vi "Labview_Voltage_Logger_All_Sensors.vi"() -> ()   [LabVIEW 2018]
doc: "I. Description:\nThis example demonstrates how to input a single Current reading on an Analog Input Channel.\n\nII. Instructions for Running:\n1. Select the Physical Channel to correspond to where your signal is input on the DAQ Device.\n2. Enter the Minimum and Maximum Current Range.\nNote: For better accuracy try to match the Input Range to the expected current level of the measured signal.\n3. Enter in the parameters of your current shunt resistor. The shunt resistor location will usually be \"External\" unless you are using an SCXI current input terminal block or SCC current input module. The shunt resistor value must correspond to the shunt resistor that you are using, and is specified in ohms. If you are using an SCXI current input terminal block or SCC current input module, you must select \"Internal\" for the shunt resistor location. \n \nIII. Block Diagram Steps:\n1. Create an Analog Input Current Channel.\n2. Use the Read VI to Acquire 1 Sample on 1 Channel on the Data Acquisition Card. \n3. Call the Clear Task VI to clear the Task. \n4. Use the popup dialog box to display an error if any. \n\nIV. I/O Connections Overview:\nMake sure your signal input terminal matches the physical channel I/O control. If you are using an external shunt resistor, make sure to hook it up in parallel with the current signal you are trying to measure."
uses:
  <vilib>/Utility/error.llb/DialogType.ctl
  <vilib>/DAQmx/read.llb/DAQmx Read (Analog DBL 1Chan 1Samp).vi
  <vilib>/DAQmx/create/channels.llb/DAQmx Create Channel (AI-Voltage-Basic).vi
  <vilib>/DAQmx/miscellaneous.llb/DAQmx Fill In Error Info.vi
panel:
  out "date/time string":string
  in  "input terminal config":i32(ring)=10106 items=["Default"=-1, "RSE"=10083, "NRSE"=10078, "Differential"=10106, "Pseudodifferential"=12529]
  in  "Durafet & DirecTemp  Spreadsheet":bool
  in  "MSFET 208 Spreadsheet":bool
  in  "MSFET 202  Spreadsheet":bool
  in  "Physical Channel 6":tag="Dev1/ai2"
  out "Ch. 3":dbl(graph)=1.4978875216444314
  in  "?":bool
  out "MS 208 Temp":dbl=nan
  out "MS 202 temp":dbl=nan
  in  "?":bool
  in  "Physical Channel 11":tag="Dev1/ai7"
  out "Ch. 8":dbl(graph)=0.8511440075618667
  in  "?":bool
  in  "Physical Channel 10":tag="Dev1/ai6"
  out "Ch. 7":dbl(graph)=0.7196247243240289
  out "DF Temp":dbl=64.59754863433032 format="%.5f"
  out "pH 3":dbl=5.329485940181883 format="%.5f"
  out "pH 2":dbl=nan format="%.5f"
  out "pH":dbl=nan format="%.5f"
  in  "Sensor in":string(combo)="DuraFET"
  out "Std dev":dbl=0.023605620391285137 format="%.5f"
  out "Voltage":dbl=0.16091888454936415 format="%.5f"
  out "Std dev":dbl=0.0006550750816912838 format="%.5f"
  out "Voltage":dbl=0.12185794600876779 format="%.5f"
  in  "?":bool
  in  "Physical Channel 9":tag="Dev1/ai5"
  out "Ch. 6":dbl(graph)=0.19601783529867856
  in  "?":bool=TRUE
  in  "?":tag="Dev1/ai4"
  out "Plot":dbl(graph)=0.12072360061828691
  out "DirecTemp":string="23.310"
  out "Ch. 4":dbl(graph)=1.780653601790566
  in  "Sensor 2":string(combo)="MSFET 208"
  in  "Sensor":string(combo)="MSFET 202"
  in  "MSFET 208":path=path "C:/Users/Garrett/Google Drive/Documents/Martz Lab/Sensors/pH_Voltages208.csv"
  in  "?":bool
  out "Run Number":i32=15
  out "Ch. 2":dbl(graph)=1.7425130298801692
  out "Ch. 1":dbl(graph)=1.5015042938814973
  in  "MSFET 202":path=path "C:/Users/Garrett/Google Drive/Documents/Martz Lab/Sensors/pH_Voltages202.csv"
  in  "# for avg.":i32=10
  in  "?":bool
  in  "?":bool
  in  "?":bool
  in  "Physical Channel 7":tag="Dev1/ai3"
  out "Std dev":dbl=nan format="%.5f"
  out "Voltage":dbl=nan format="%.5f"
  out "Std dev":dbl=nan format="%.5f"
  out "Std dev":dbl=nan format="%.5f"
  out "Std dev":dbl=nan format="%.6f"
  in  "Max Voltage":dbl=1.0 format="%0.3f"
  in  "Min Voltage":dbl=-1.0 format="%0.3f"
  in  "Physical Channel 5":tag="Dev1/ai1"
  out "Voltage":dbl=nan format="%.5f"
  out "Voltage":dbl=nan format="%.5f"
  in  "Physical Channel 4":tag="Dev1/ai0"
  out "Voltage":dbl=nan format="%.6f"
  in  "For DuraFET":path=path "C:/Users/Garrett/Google Drive/Documents/Martz Lab/Sensors/pH_VoltagesDurafet.csv"
  # "OUTPUTS"
  # "INPUTS"
  # "Min Voltage"
  # "Max Voltage"
  # "Amount of meas. to avg. for data point"
  # "MSFET 202"
  # "MSFET 208"
  # "REF Voltage"
  # "pH Voltage"
  # "REF Voltage"
  # "pH Voltage"
  # "pH Voltage"
  # "Temp Voltage"
  # "Temp Voltage"
  # "Temp Voltage"
  # "+ AI0 -"
  # "+ AI1 -"
  # "+ AI2 -"
  # "+ AI3 -"
  # "+ AI4 -"
  # "+ AI5-"
  # "+ AI6-"
  # "+ AI7-"
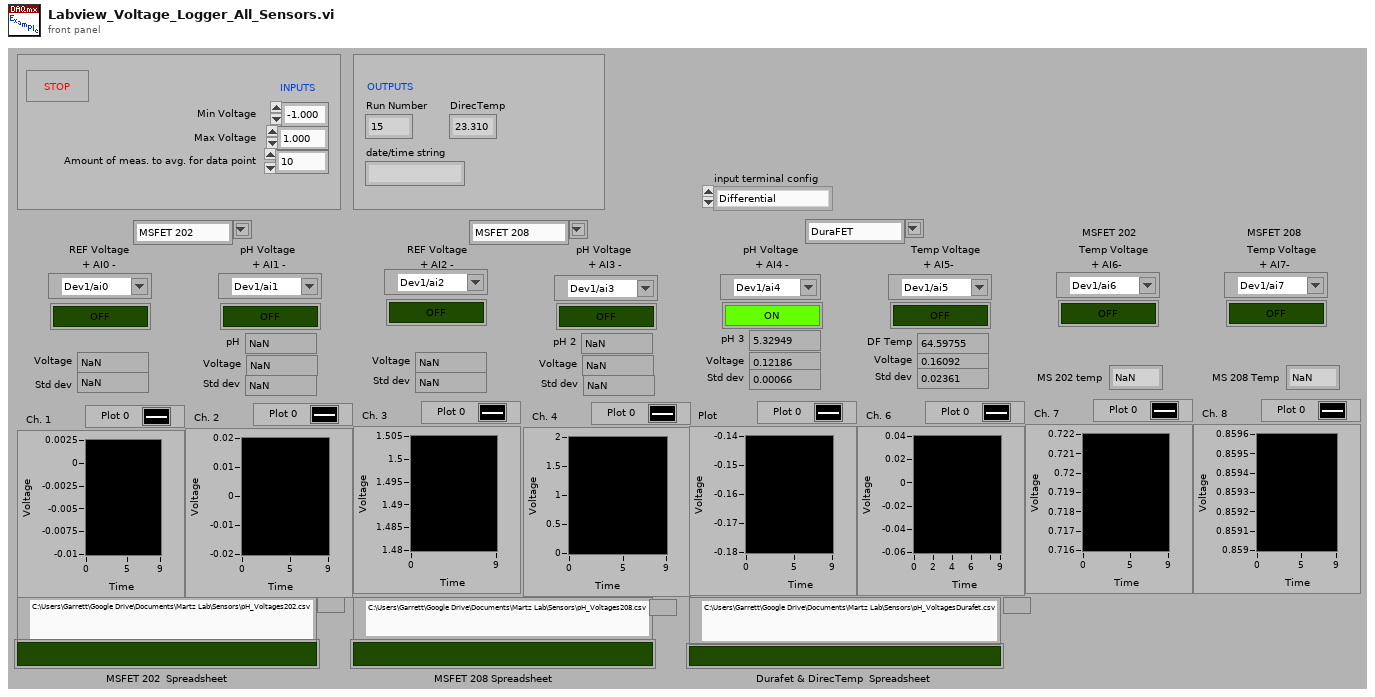
[diagram p1: front panel]
types:
  T1 = typedef "DialogType.ctl" = u16
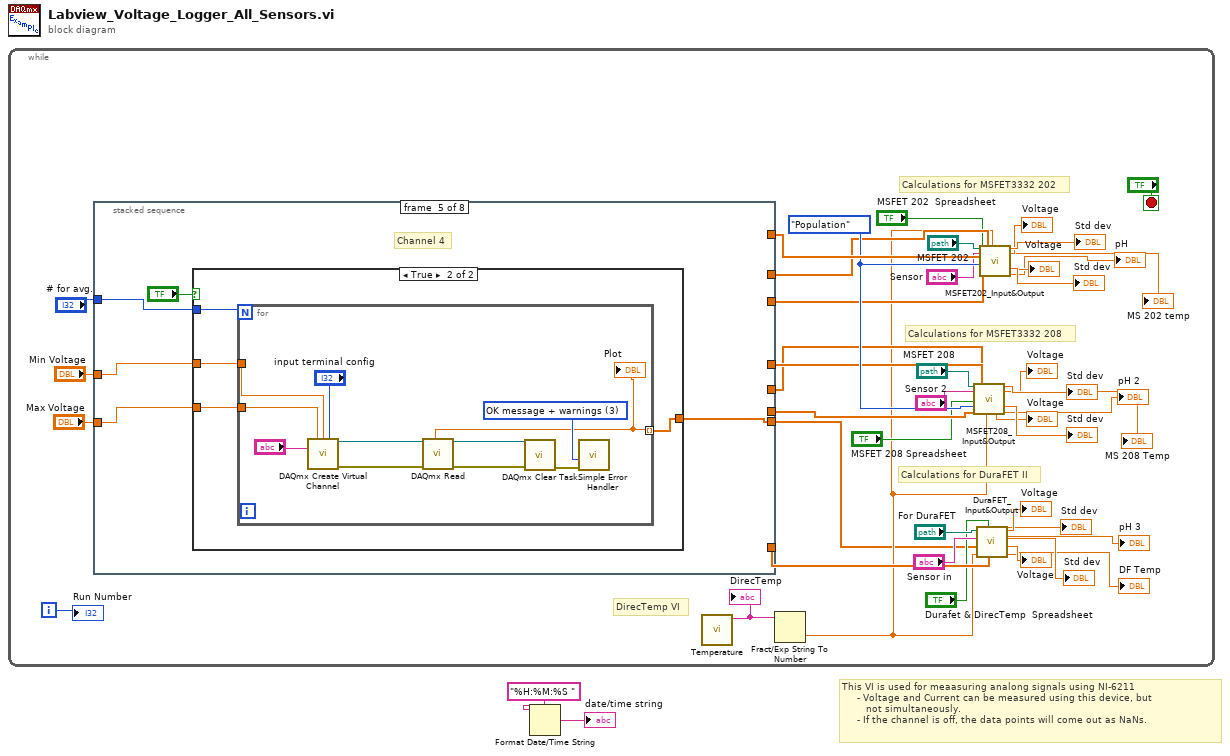
[diagram p0: block diagram]
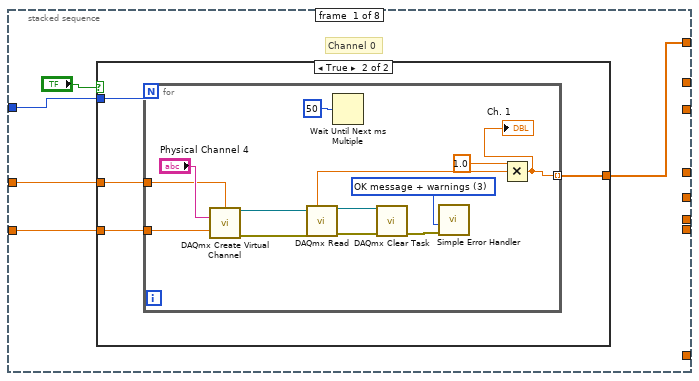
[diagram p2: hidden frame]
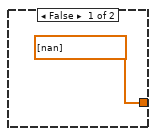
[diagram p3: hidden frame]
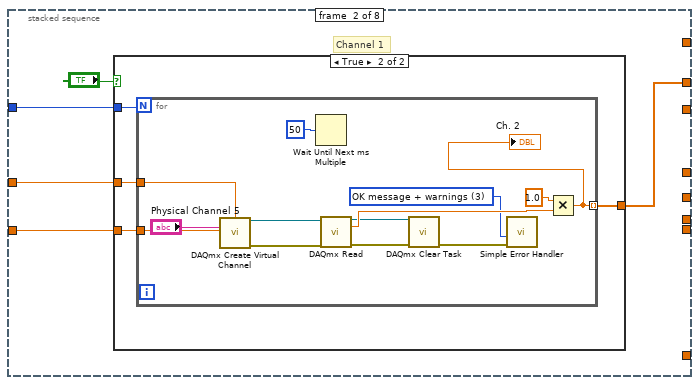
[diagram p4: hidden frame]
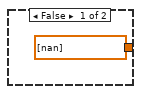
[diagram p5: hidden frame]
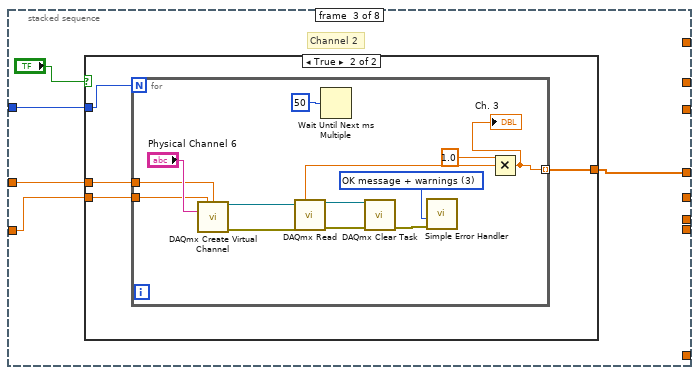
[diagram p6: hidden frame]
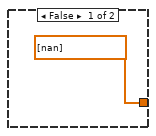
[diagram p7: hidden frame]
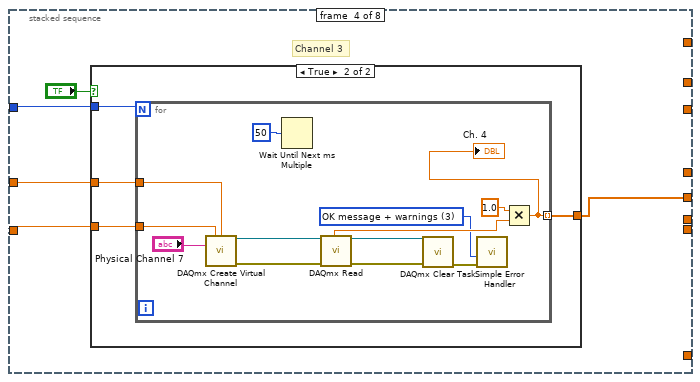
[diagram p8: hidden frame]
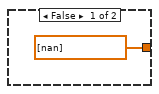
[diagram p9: hidden frame]
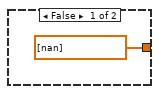
[diagram p10: hidden frame]
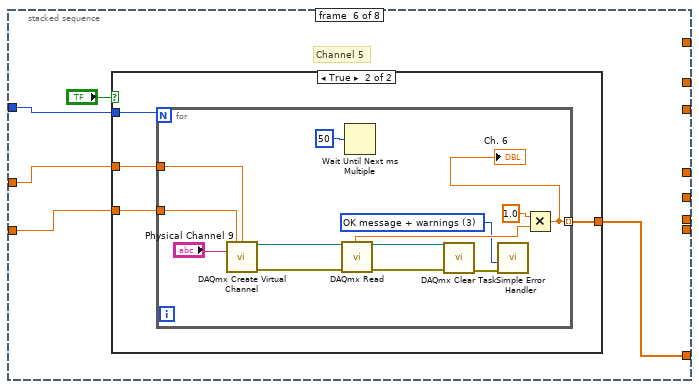
[diagram p11: hidden frame]
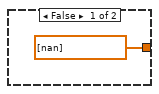
[diagram p12: hidden frame]
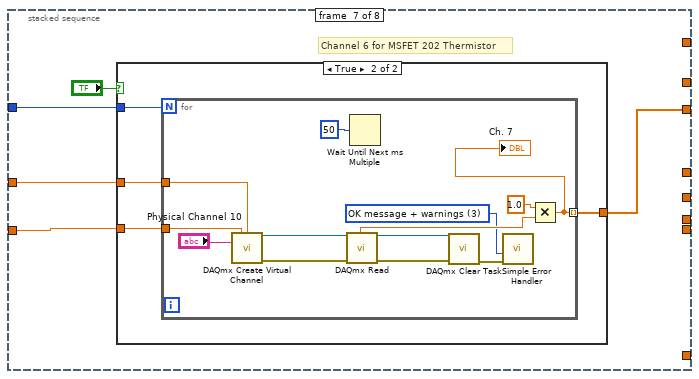
[diagram p13: hidden frame]
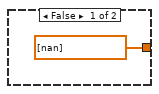
[diagram p14: hidden frame]
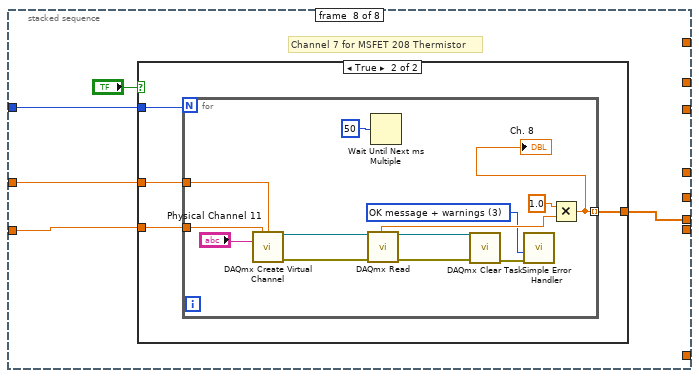
[diagram p15: hidden frame]
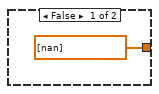
[diagram p16: hidden frame]
diagram:
  # "This VI is used for meaasuring analong signals using NI-6211\n     - Voltage and Current can be measured using this device, but \n        not simultaneously. \n     - If the channel is off, the data points will come out as NaNs."
  n1 = while {
    i -> [w41]
    stop <- "?" stop-if-true
    w44 = enum16{"Sample", "Population"}."Population" ("Weighting (Sample)")
    # "DirecTemp VI"
    # "Calculations for DuraFET II"
    # "Calculations for MSFET3332 208"
    # "Calculations for MSFET3332 202"
    n2 = stacked-sequence {
      tunnel: [_ w73 _ _ _ _ _ _] -> w42
      tunnel: [w49 _ _ _ _ _ _ _] -> w45
      tunnel: "Min Voltage" -> [w48 w71 w94 w117 w141 w161 w184 w207]
      tunnel: "Max Voltage" -> [w47 w70 w93 w116 w140 w160 w183 w206]
      tunnel: "# for avg." -> [w46 w69 w95 w118 w138 w162 w185 w208]
      tunnel: [_ _ _ _ _ w159 _ _] -> w24
      tunnel: [_ _ _ w115 _ _ _ _] -> w9
      tunnel: [_ _ _ _ _ _ w182 _] -> w12
      tunnel: [_ _ w92 _ _ _ _ _] -> w10
      tunnel: [_ _ _ _ _ _ _ w205] -> w8
      tunnel: [_ _ _ _ w139 _ _ _] -> w3
      frame #0 {
        # "Channel 0"
        n3 = case shown="True" "?" {
          tunnel: [dbl[] [nan] w55] -> w49
          tunnel: w48 -> [_ w54]
          tunnel: w47 -> [_ w53]
          tunnel: w46 -> [_ w52]
          frame False {
          }
          frame True {
            n4 = for {
              N: w52 -> [_]
              tunnel: [w60] -> w55 mode=indexing
              tunnel: w54 -> [w57]
              tunnel: w53 -> [w56]
              w63 = T1 3 items=["no dialog", "OK message", "continue or stop message", "OK message + warnings", "continue/stop + warnings"] ("type of dialog (OK msg:1)")
              n5 = call-poly <vilib>:"DAQmx Create Virtual Channel.vi"("maximum value"=w56, "minimum value"=w57, "physical channels"="Physical Channel 4") -> ("task out"=w59:refnum<k21>, "error out"=w58:errorcluster)  [unwired: 11 in]
              n6 = call-poly <vilib>:"DAQmx Read.vi"("task/channels in"=w59, "error in"=w58) -> ("task out"=w64:refnum<k21>, "data"=w68:dbl, "error out"=w65:errorcluster)  [unwired: 11 in]
              n7 = Wait Until Next ms Multiple(millisecond multiple=u32 50) -> ()  [unwired: 1 out]
              n8 = call <vilib>:"DAQmx Clear Task.vi"("task in"=w64, "error in"=w65) -> ("error out"=w66:errorcluster)  [unwired: 13 in]
              n9 = call <vilib>:"Simple Error Handler.vi"("type of dialog (OK msg:1)"=w63, "error in (no error)"=w66) -> ()  [unwired: 3 in, 5 out]
              n10 = Multiply(x=1.0, y=w68) -> (x*y=w60:dbl)
              "Ch. 1" <- w60
            }
          }
        }
      }
      frame #1 {
        # "Channel 1"
        n11 = case shown="True" "?" {
          tunnel: [dbl[] [nan] w78] -> w73
          tunnel: w71 -> [_ w77]
          tunnel: w70 -> [_ w76]
          tunnel: w69 -> [_ w75]
          frame False {
          }
          frame True {
            n12 = for {
              N: w75 -> [_]
              tunnel: [w83] -> w78 mode=indexing
              tunnel: w77 -> [w80]
              tunnel: w76 -> [w79]
              w86 = T1 3 items=["no dialog", "OK message", "continue or stop message", "OK message + warnings", "continue/stop + warnings"] ("type of dialog (OK msg:1)")
              n13 = call-poly <vilib>:"DAQmx Create Virtual Channel.vi"("maximum value"=w79, "minimum value"=w80, "physical channels"="Physical Channel 5") -> ("task out"=w82:refnum<k21>, "error out"=w81:errorcluster)  [unwired: 11 in]
              n14 = Wait Until Next ms Multiple(millisecond multiple=u32 50) -> ()  [unwired: 1 out]
              n15 = call-poly <vilib>:"DAQmx Read.vi"("task/channels in"=w82, "error in"=w81) -> ("task out"=w87:refnum<k21>, "data"=w91:dbl, "error out"=w88:errorcluster)  [unwired: 11 in]
              n16 = call <vilib>:"DAQmx Clear Task.vi"("task in"=w87, "error in"=w88) -> ("error out"=w89:errorcluster)  [unwired: 13 in]
              n17 = call <vilib>:"Simple Error Handler.vi"("type of dialog (OK msg:1)"=w86, "error in (no error)"=w89) -> ()  [unwired: 3 in, 5 out]
              n18 = Multiply(x=1.0, y=w91) -> (x*y=w83:dbl)
              "Ch. 2" <- w83
            }
          }
        }
      }
      frame #2 {
        # "Channel 2"
        n19 = case shown="True" "?" {
          tunnel: [dbl[] [nan] w101] -> w92
          tunnel: w95 -> [_ w100]
          tunnel: w94 -> [_ w99]
          tunnel: w93 -> [_ w98]
          frame False {
          }
          frame True {
            n20 = for {
              N: w100 -> [_]
              tunnel: [w106] -> w101 mode=indexing
              tunnel: w99 -> [w103]
              tunnel: w98 -> [w102]
              w109 = T1 3 items=["no dialog", "OK message", "continue or stop message", "OK message + warnings", "continue/stop + warnings"] ("type of dialog (OK msg:1)")
              n21 = call-poly <vilib>:"DAQmx Create Virtual Channel.vi"("maximum value"=w102, "minimum value"=w103, "physical channels"="Physical Channel 6") -> ("task out"=w105:refnum<k21>, "error out"=w104:errorcluster)  [unwired: 11 in]
              n22 = call-poly <vilib>:"DAQmx Read.vi"("task/channels in"=w105, "error in"=w104) -> ("task out"=w110:refnum<k21>, "data"=w114:dbl, "error out"=w111:errorcluster)  [unwired: 11 in]
              n23 = Wait Until Next ms Multiple(millisecond multiple=u32 50) -> ()  [unwired: 1 out]
              n24 = call <vilib>:"DAQmx Clear Task.vi"("task in"=w110, "error in"=w111) -> ("error out"=w112:errorcluster)  [unwired: 13 in]
              n25 = call <vilib>:"Simple Error Handler.vi"("type of dialog (OK msg:1)"=w109, "error in (no error)"=w112) -> ()  [unwired: 3 in, 5 out]
              n26 = Multiply(x=1.0, y=w114) -> (x*y=w106:dbl)
              "Ch. 3" <- w106
            }
          }
        }
      }
      frame #3 {
        # "Channel 3"
        n27 = case shown="True" "?" {
          tunnel: [dbl[] [nan] w124] -> w115
          tunnel: w118 -> [_ w123]
          tunnel: w117 -> [_ w122]
          tunnel: w116 -> [_ w121]
          frame False {
          }
          frame True {
            n28 = for {
              N: w123 -> [_]
              tunnel: [w129] -> w124 mode=indexing
              tunnel: w122 -> [w126]
              tunnel: w121 -> [w125]
              w132 = T1 3 items=["no dialog", "OK message", "continue or stop message", "OK message + warnings", "continue/stop + warnings"] ("type of dialog (OK msg:1)")
              n29 = call-poly <vilib>:"DAQmx Create Virtual Channel.vi"("maximum value"=w125, "minimum value"=w126, "physical channels"="Physical Channel 7") -> ("task out"=w128:refnum<k21>, "error out"=w127:errorcluster)  [unwired: 11 in]
              n30 = Wait Until Next ms Multiple(millisecond multiple=u32 50) -> ()  [unwired: 1 out]
              n31 = call-poly <vilib>:"DAQmx Read.vi"("task/channels in"=w128, "error in"=w127) -> ("task out"=w133:refnum<k21>, "data"=w137:dbl, "error out"=w134:errorcluster)  [unwired: 11 in]
              n32 = call <vilib>:"DAQmx Clear Task.vi"("task in"=w133, "error in"=w134) -> ("error out"=w135:errorcluster)  [unwired: 13 in]
              n33 = call <vilib>:"Simple Error Handler.vi"("type of dialog (OK msg:1)"=w132, "error in (no error)"=w135) -> ()  [unwired: 3 in, 5 out]
              n34 = Multiply(x=1.0, y=w137) -> (x*y=w129:dbl)
              "Ch. 4" <- w129
            }
          }
        }
      }
      frame #4 {
        # "Channel 4"
        n35 = case shown="True" "?" {
          tunnel: [dbl[] [nan] w144] -> w139
          tunnel: w138 -> [_ w147]
          tunnel: w141 -> [_ w146]
          tunnel: w140 -> [_ w145]
          frame False {
          }
          frame True {
            n36 = for {
              N: w147 -> [_]
              tunnel: w146 -> [w151]
              tunnel: w145 -> [w150]
              tunnel: [w148] -> w144 mode=indexing
              w155 = T1 3 items=["no dialog", "OK message", "continue or stop message", "OK message + warnings", "continue/stop + warnings"] ("type of dialog (OK msg:1)")
              n37 = call-poly <vilib>:"DAQmx Create Virtual Channel.vi"("maximum value"=w150, "minimum value"=w151, "input terminal configuration"="input terminal config", "physical channels"="?") -> ("task out"=w153:refnum<k21>, "error out"=w152:errorcluster)  [unwired: 10 in]
              n38 = call-poly <vilib>:"DAQmx Read.vi"("task/channels in"=w153, "error in"=w152) -> ("task out"=w156:refnum<k21>, "data"=w148:dbl, "error out"=w157:errorcluster)  [unwired: 11 in]
              "Plot" <- w148
              n39 = call <vilib>:"DAQmx Clear Task.vi"("task in"=w156, "error in"=w157) -> ("error out"=w158:errorcluster)  [unwired: 13 in]
              n40 = call <vilib>:"Simple Error Handler.vi"("type of dialog (OK msg:1)"=w155, "error in (no error)"=w158) -> ()  [unwired: 3 in, 5 out]
            }
          }
        }
      }
      frame #5 {
        # "Channel 5"
        n41 = case shown="True" "?" {
          tunnel: [dbl[] [nan] w168] -> w159
          tunnel: w162 -> [_ w167]
          tunnel: w161 -> [_ w166]
          tunnel: w160 -> [_ w165]
          frame False {
          }
          frame True {
            n42 = for {
              N: w167 -> [_]
              tunnel: [w173] -> w168 mode=indexing
              tunnel: w166 -> [w170]
              tunnel: w165 -> [w169]
              w176 = T1 3 items=["no dialog", "OK message", "continue or stop message", "OK message + warnings", "continue/stop + warnings"] ("type of dialog (OK msg:1)")
              n43 = call-poly <vilib>:"DAQmx Create Virtual Channel.vi"("maximum value"=w169, "minimum value"=w170, "physical channels"="Physical Channel 9") -> ("task out"=w172:refnum<k21>, "error out"=w171:errorcluster)  [unwired: 11 in]
              n44 = call-poly <vilib>:"DAQmx Read.vi"("task/channels in"=w172, "error in"=w171) -> ("task out"=w177:refnum<k21>, "data"=w181:dbl, "error out"=w178:errorcluster)  [unwired: 11 in]
              n45 = Wait Until Next ms Multiple(millisecond multiple=u32 50) -> ()  [unwired: 1 out]
              n46 = call <vilib>:"DAQmx Clear Task.vi"("task in"=w177, "error in"=w178) -> ("error out"=w179:errorcluster)  [unwired: 13 in]
              n47 = call <vilib>:"Simple Error Handler.vi"("type of dialog (OK msg:1)"=w176, "error in (no error)"=w179) -> ()  [unwired: 3 in, 5 out]
              n48 = Multiply(x=1.0, y=w181) -> (x*y=w173:dbl)
              "Ch. 6" <- w173
            }
          }
        }
      }
      frame #6 {
        # "Channel 6 for MSFET 202 Thermistor"
        n49 = case shown="True" "?" {
          tunnel: [dbl[] [nan] w191] -> w182
          tunnel: w185 -> [_ w190]
          tunnel: w184 -> [_ w189]
          tunnel: w183 -> [_ w188]
          frame False {
          }
          frame True {
            n50 = for {
              N: w190 -> [_]
              tunnel: [w196] -> w191 mode=indexing
              tunnel: w189 -> [w193]
              tunnel: w188 -> [w192]
              w199 = T1 3 items=["no dialog", "OK message", "continue or stop message", "OK message + warnings", "continue/stop + warnings"] ("type of dialog (OK msg:1)")
              n51 = call-poly <vilib>:"DAQmx Create Virtual Channel.vi"("maximum value"=w192, "minimum value"=w193, "physical channels"="Physical Channel 10") -> ("task out"=w195:refnum<k21>, "error out"=w194:errorcluster)  [unwired: 11 in]
              n52 = call-poly <vilib>:"DAQmx Read.vi"("task/channels in"=w195, "error in"=w194) -> ("task out"=w200:refnum<k21>, "data"=w204:dbl, "error out"=w201:errorcluster)  [unwired: 11 in]
              n53 = Wait Until Next ms Multiple(millisecond multiple=u32 50) -> ()  [unwired: 1 out]
              n54 = call <vilib>:"DAQmx Clear Task.vi"("task in"=w200, "error in"=w201) -> ("error out"=w202:errorcluster)  [unwired: 13 in]
              n55 = call <vilib>:"Simple Error Handler.vi"("type of dialog (OK msg:1)"=w199, "error in (no error)"=w202) -> ()  [unwired: 3 in, 5 out]
              n56 = Multiply(x=1.0, y=w204) -> (x*y=w196:dbl)
              "Ch. 7" <- w196
            }
          }
        }
      }
      frame #7 {
        # "Channel 7 for MSFET 208 Thermistor"
        n57 = case shown="True" "?" {
          tunnel: [dbl[] [nan] w214] -> w205
          tunnel: w208 -> [_ w213]
          tunnel: w207 -> [_ w212]
          tunnel: w206 -> [_ w211]
          frame False {
          }
          frame True {
            n58 = for {
              N: w213 -> [_]
              tunnel: [w219] -> w214 mode=indexing
              tunnel: w212 -> [w216]
              tunnel: w211 -> [w215]
              w222 = T1 3 items=["no dialog", "OK message", "continue or stop message", "OK message + warnings", "continue/stop + warnings"] ("type of dialog (OK msg:1)")
              n59 = call-poly <vilib>:"DAQmx Create Virtual Channel.vi"("maximum value"=w215, "minimum value"=w216, "physical channels"="Physical Channel 11") -> ("task out"=w218:refnum<k21>, "error out"=w217:errorcluster)  [unwired: 11 in]
              n60 = call-poly <vilib>:"DAQmx Read.vi"("task/channels in"=w218, "error in"=w217) -> ("task out"=w223:refnum<k21>, "data"=w227:dbl, "error out"=w224:errorcluster)  [unwired: 11 in]
              n61 = Wait Until Next ms Multiple(millisecond multiple=u32 50) -> ()  [unwired: 1 out]
              n62 = call <vilib>:"DAQmx Clear Task.vi"("task in"=w223, "error in"=w224) -> ("error out"=w225:errorcluster)  [unwired: 13 in]
              n63 = call <vilib>:"Simple Error Handler.vi"("type of dialog (OK msg:1)"=w222, "error in (no error)"=w225) -> ()  [unwired: 3 in, 5 out]
              n64 = Multiply(x=1.0, y=w227) -> (x*y=w219:dbl)
              "Ch. 8" <- w219
            }
          }
        }
      }
    }
    n65 = call "Temperature.vi"() -> ("read buffer"=w14:string)  [unwired: 11 in]
    "DirecTemp" <- w14
    n66 = Fract/Exp String To Number(string=w14) -> (number=w4:dbl)  [unwired: 3 in, 1 out]
    n67 = call "MSFET208_Input&Output.vi"("Data Saved in"="MSFET 208", "Sensor in"="Sensor 2", "Boolean"="MSFET 208 Spreadsheet", "Weighting (Sample)"=w44, "Temp Voltage"=w8, "ISFET Voltage"=w9, "REF voltage"=w10, "DirecTemp"=w4) -> ("MS 208 Temp"=→"MS 208 Temp":dbl, "Mean3"=→"Voltage":dbl, "std2"=→"Std dev":dbl, "Mean2"=→"Voltage":dbl, "std3"=→"Std dev":dbl, "pHint"=→"pH 2":dbl)  [unwired: 6 in]
    n68 = call "DuraFET_Input&Output.vi"("Temp Voltage"=w24, "Write ro Spreadsheet?"="Durafet & DirecTemp  Spreadsheet", "DirecTemp"=w4, "pH voltage"=w3, "Sensor in"="Sensor in", "Spec. On Front Panel"="For DuraFET") -> ("DuraFET Temp"=→"DF Temp":dbl, "Mean5"=→"Voltage":dbl, "std5"=→"Std dev":dbl, "pH voltage mean"=→"Voltage":dbl, "pH voltage stdev"=→"Std dev":dbl, "pHint"=→"pH 3":dbl)
    n69 = call "MSFET202_Input&Output.vi"("Data Saved"="MSFET 202", "Sensor"="Sensor", "Boolean"="MSFET 202  Spreadsheet", "Weighting (Sample)"=w44, "Temp Voltage"=w12, "ISFET Voltage\\"=w42, "REF Voltage"=w45, "DirecTemp"=w4) -> ("Temperature (C)"=→"MS 202 temp":dbl, "Mean1"=→"Voltage":dbl, "std0"=→"Std dev":dbl, "Mean0"=→"Voltage":dbl, "std1"=→"Std dev":dbl, "pHint"=→"pH":dbl)  [unwired: 6 in]
    "Run Number" <- w41
  }
  n70 = Format Date/Time String(time format string (%c)="%H:%M:%S ") -> (date/time string=→"date/time string":string)  [unwired: 2 in]
